vi "Target3.1.vi"   [LabVIEW 2025]
uses:
  <vilib>/rvi/DataTransferAndStorage/Container/XNode/niFpgaContainer.xnode
  <vilib>/rvi/interface/RandomDataEmulation/nirviRandomDataFpgaReadWriteTemplate.vi
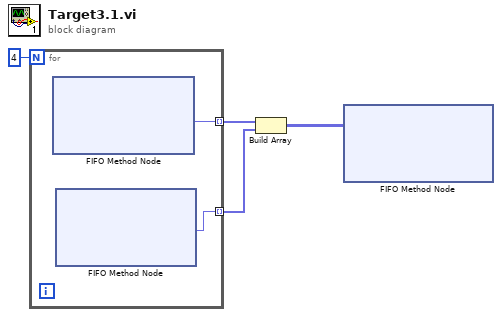
[diagram p0: block diagram]
diagram:
  n1 = for {
    N: 4 -> [_]
    tunnel: [w6] -> w3 mode=indexing
    tunnel: [w5] -> w2 mode=indexing
    n2 = xnode ("FIFO Method Node")() -> ("Element"=w5:fxp<+/-,32,16>)  [unwired: 2 in, 2 out]
    n3 = xnode ("FIFO Method Node")() -> ("Element"=w6:fxp<+/-,32,16>)  [unwired: 2 in, 2 out]
  }
  n4 = Build Array(w2, w3) -> (w1:fxp<+/-,32,16>[][])
  n5 = xnode ("FIFO Method Node")("Element"=w1) -> ()  [unwired: 2 in, 2 out]
